vi "Read VAR.vi"(5 "Flow Meter DevID":i32=1, 7 "Timeout (ms)":u32, 8 "error in":errorcluster, 10 "Variable to Read":T1, 11 "VISA resource name":refnum<visa-resource-name>) -> (0 "error out":errorcluster, 1 "Read Buffer":string, 3 "VISA resource name out":refnum<visa-resource-name>)   [LabVIEW 2010, in "FEM-03.lvlib"]
uses:
  FEM-03.lvlib
  Private/Controls/Variable List.ctl
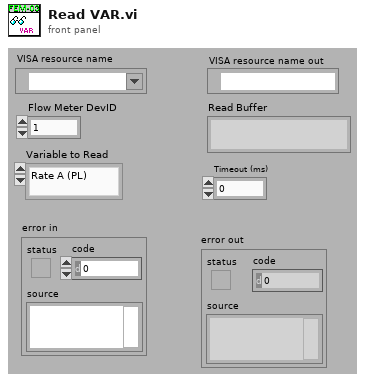
[diagram p1: front panel]
types:
  T1 = typedef "FEM-03.lvlib/Variable List.ctl" = enum16{"Rate A (PL)", "Rate A (GT)", "Job Total A", "Grand Total A", "A-KFR for Rate", "A-KFR decimal point location", "A-KFT for Total", "A-KFT decimal point location ", "A-Rate Engineering Units", "A-Total Engineering units", "A-Flow Direction", "Rate B (PL)", "Rate B (GT)", "Job Total B", "Grand Total B", "B-KFR for Rate", "B-KFR deciminal point location", "B-Rate Engineering units", "B-KFT for Total", "B-KFT decimal point location", "B-Total Engineering units", "Limit 1 Mode", "Limit1", "Margin 1 for rate limit", "Limit 2 Mode", "Limit2", "Margin 2 for rate limit", "Milli-amps Offset", "Milli-amps Out", "Analog Out Mode", "Serial Speed", "Unit Number", "Serial RESET TOTAL", "Update EEPROM", "Relay Override", "FORCE mA Output"}
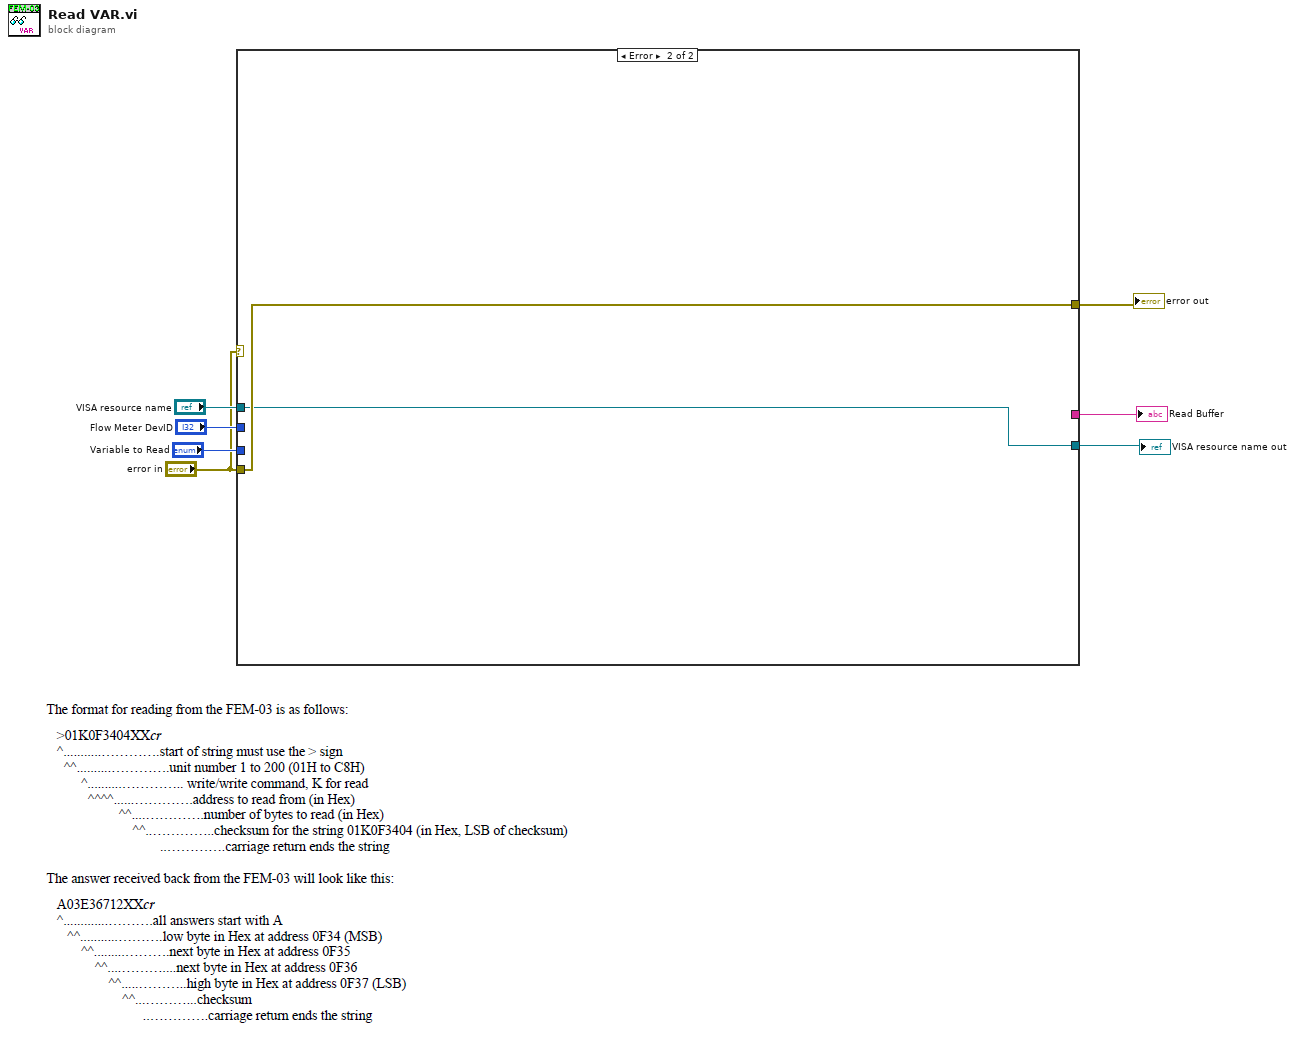
[diagram p0: block diagram]
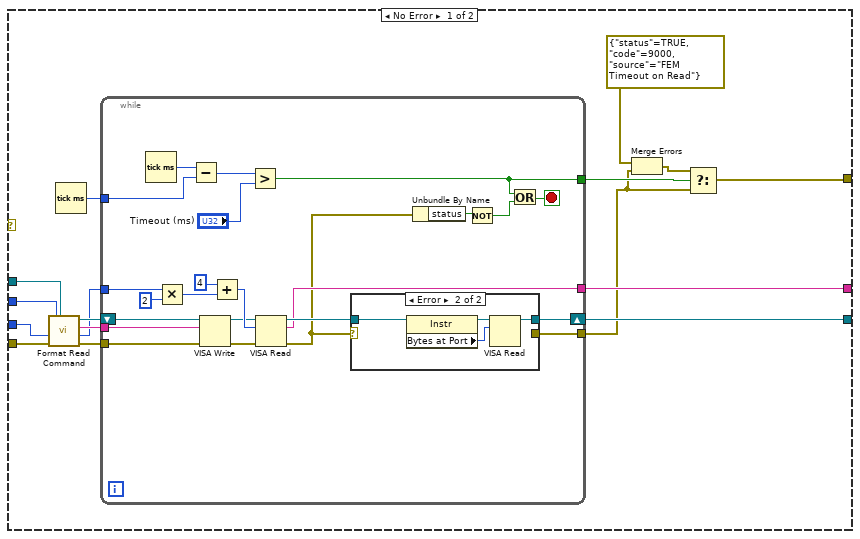
[diagram p2: hidden frame]
diagram:
  n1 = case shown="Error" "error in" {
    tunnel: "Flow Meter DevID" -> [w23 _]
    tunnel: "VISA resource name" -> [w19 w53]
    tunnel: "error in" -> [w18 w54]
    tunnel: [w16 _] -> w5
    tunnel: [w15 w53] -> w4
    tunnel: "Variable to Read" -> [w13 _]
    tunnel: [w11 w54] -> w2
    frame No Error {
      n2 = call "Format Read Command.vi"("error in"=w18, "Variable to Read"=w13, "Flow Meter DevID"=w23, "VISA resource name"=w19) -> ("error out"=w22:errorcluster, "Length Bytes (Dec)"=w17:i32, "Command String with Checksum"=w20:string, "VISA resource name out"=w21:refnum<visa-resource-name>)
      n3 = Tick Count (ms)() -> (millisecond timer value=w14:u32)
      n4 = while {
        tunnel: w22 -> [w46]
        tunnel: w20 -> [w44]
        tunnel: w17 -> [w43]
        shift-right: [w35] -> w15
        shift-left: w21 -> [w45]
        tunnel: [w34] -> w9
        tunnel: [w33] -> w16
        tunnel: w14 -> [w31]
        tunnel: [w25] -> w12
        stop <- w26 stop-if-true
        n5 = Tick Count (ms)() -> (millisecond timer value=w32:u32)
        n6 = Multiply(x=w43, y=2) -> (x*y=w41:i32)
        n7 = Subtract(x=w32, y=w31) -> (x-y=w29:u32)
        n8 = VISA Write(VISA resource name=w45, write buffer=w44, error in (no error)=w46) -> (VISA resource name out=w38:refnum<visa-resource-name>, error out=w37:errorcluster)  [unwired: 1 out]
        n9 = Add(x=4, y=w41) -> (x+y=w39:i32)
        n10 = Greater?(x=w29, y="Timeout (ms)") -> (0:w25:bool)
        n11 = VISA Read(VISA resource name=w38, byte count=w39, error in (no error)=w37) -> (VISA resource name out=w36:refnum<visa-resource-name>, read buffer=w33:string, error out=w24:errorcluster)  [unwired: 1 out]
        n12 = case shown="Error" w24 {
          selector: w24 -> [w48 _]
          tunnel: w36 -> [w47 w52]
          tunnel: [w47 w49] -> w35
          tunnel: [w48 _] -> w34
          frame No Error {
          }
          frame Error {
            n13 = property class="Instr"(reference=w52) -> (reference out=w51:refnum<visa-resource-name>, "Bytes at Port"=w50:u32)  [unwired: 1 in, 1 out]
            n14 = VISA Read(VISA resource name=w51, byte count=w50) -> (VISA resource name out=w49:refnum<visa-resource-name>)  [unwired: 1 in, 3 out]
          }
        }
        n15 = Unbundle By Name(w24) -> ("status"=w28:bool)
        n16 = Not(x=w28) -> (.not. x?=w27:bool)
        n17 = Or(x=w25, y=w27) -> (x .or. y?=w26:bool)
      }
      n18 = Merge Errors(errorcluster {"status"=TRUE, "code"=9000, "source"="FEM Timeout on Read"} ("error out"), w9) -> (w8:errorcluster)
      n19 = Select(t=w8, s=w12, f=w9) -> (s? t:f=w11:errorcluster)
    }
    frame Error {
    }
  }
  "Read Buffer" <- w5
  "VISA resource name out" <- w4
  "error out" <- w2
